vi "Write Configuration Settings File.vi"(8 "error in (no error)":errorcluster, 11 "refnum":T1) -> (0 "error out":errorcluster, 3 "refnum out":T1)   [LabVIEW 2017]
doc: "Illustrates how to create and write a configuration settings file.\n\nInstructions:\nEnter values in the controls on the front panel then click on the Run Arrow.\nTo read the file, run Read Configuration Settings File.vi located in the file\\config.llb."
uses:
  <vilib>/Utility/config.llb/Config Data RefNum.ctl
  Boiler System Globals.vi
  <vilib>/Utility/config.llb/Write Key (Double).vi
  <vilib>/Utility/config.llb/Write Key (U32).vi
  <vilib>/Utility/config.llb/NI_LVConfig.lvlib
panel:
  in  "Pilot Decrement (ms)":u32=50
  in  "Pilot Increment (ms)":u32=100
  in  "Flame Threshold":u32=30
  in  "Purge Time":u32=2
  in  "Fuel Control Valve Minimum":dbl=10.0
  in  "Fuel Control Valve Maximum":dbl=75.0
  # "Instructions:\nEnter values in the controls below, then click on the Run arrow.  The VI will write these values into the selected configuration settings file."
  # "MHL"
  # "Controller"
  # "Boiler"
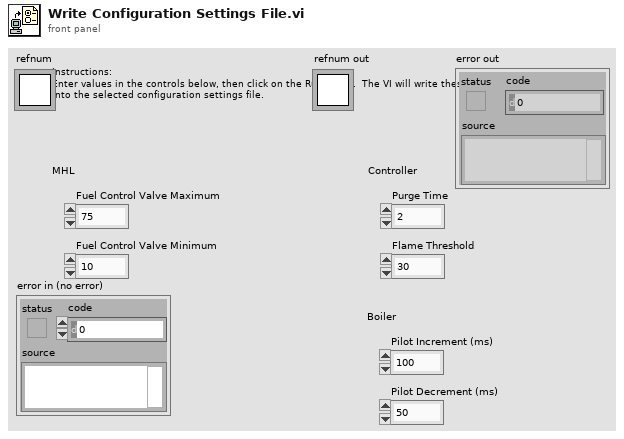
[diagram p1: front panel]
types:
  T1 = typedef "NI_LVConfig.lvlib/Config Data RefNum.ctl" = refnum<k1>
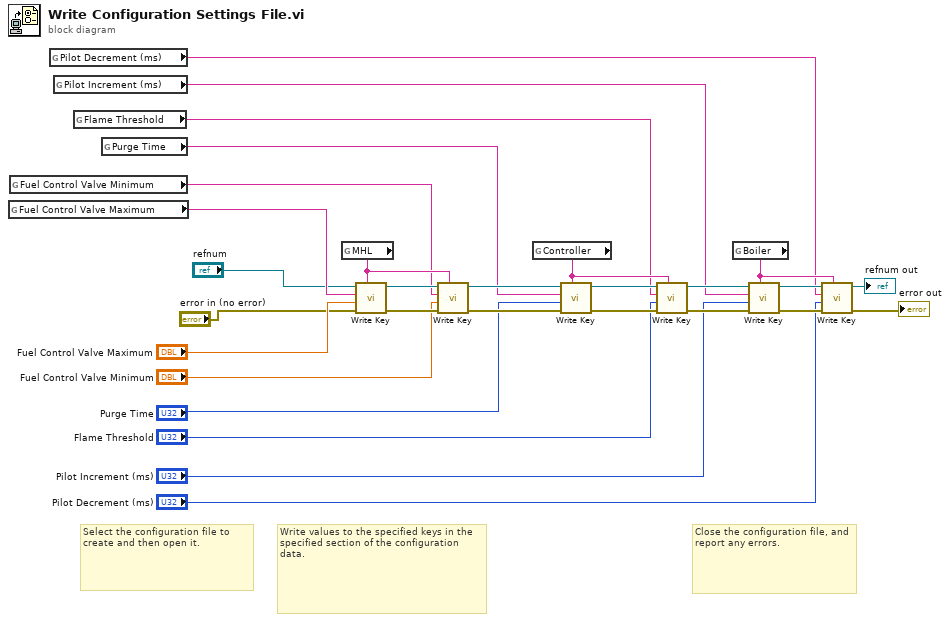
[diagram p0: block diagram]
diagram:
  # "Close the configuration file, and report any errors."
  # "Write values to the specified keys in the specified section of the configuration data."
  # "Select the configuration file to create and then open it."
  n1 = global read "Boiler System Globals.vi" "Fuel Control Valve Maximum"() -> (w29:string)
  n2 = global read "Boiler System Globals.vi" "Fuel Control Valve Minimum"() -> (w22:string)
  n3 = global read "Boiler System Globals.vi" "Pilot Decrement (ms)"() -> (w6:string)
  n4 = global read "Boiler System Globals.vi" "Pilot Increment (ms)"() -> (w7:string)
  n5 = global read "Boiler System Globals.vi" "Flame Threshold"() -> (w14:string)
  n6 = global read "Boiler System Globals.vi" "Purge Time"() -> (w19:string)
  n7 = global read "Boiler System Globals.vi" "MHL"() -> (w25:string)
  n8 = call-poly <vilib>:"Write Key.vi"("section"=w25, "error in (no error)"="error in (no error)", "value"="Fuel Control Valve Maximum", "key"=w29, "refnum"="refnum") -> ("error out"=w27:errorcluster, "refnum out"=w26:T1)  [unwired: 4 in, 1 out]
  n9 = call-poly <vilib>:"Write Key.vi"("section"=w25, "error in (no error)"=w27, "value"="Fuel Control Valve Minimum", "key"=w22, "refnum"=w26) -> ("error out"=w24:errorcluster, "refnum out"=w20:T1)  [unwired: 4 in, 1 out]
  n10 = global read "Boiler System Globals.vi" "Controller"() -> (w16:string)
  n11 = call-poly <vilib>:"Write Key.vi"("section"=w16, "error in (no error)"=w24, "value"="Purge Time", "key"=w19, "refnum"=w20) -> ("error out"=w21:errorcluster, "refnum out"=w17:T1)  [unwired: 4 in, 1 out]
  n12 = call-poly <vilib>:"Write Key.vi"("section"=w16, "error in (no error)"=w21, "value"="Flame Threshold", "key"=w14, "refnum"=w17) -> ("error out"=w10:errorcluster, "refnum out"=w9:T1)  [unwired: 4 in, 1 out]
  n13 = global read "Boiler System Globals.vi" "Boiler"() -> (w13:string)
  n14 = call-poly <vilib>:"Write Key.vi"("section"=w13, "error in (no error)"=w10, "value"="Pilot Increment (ms)", "key"=w7, "refnum"=w9) -> ("error out"=w11:errorcluster, "refnum out"=w12:T1)  [unwired: 4 in, 1 out]
  n15 = call-poly <vilib>:"Write Key.vi"("section"=w13, "error in (no error)"=w11, "value"="Pilot Decrement (ms)", "key"=w6, "refnum"=w12) -> ("error out"=→"error out":errorcluster, "refnum out"=→"refnum out":T1)  [unwired: 4 in, 1 out]
